vi "S to T - 4Port.vi"(8 "error in (no error)":errorcluster, 11 "S-par Array In":cdb[][](array[numeric])) -> (0 "error out":errorcluster, 3 "T-par Array Out":cdb[][](array[numeric]))   [LabVIEW 2020]
uses:
  <vilib>/Analysis/Matrix/Datatypes/RealMatrix.ctl
  <vilib>/Analysis/baseanly.llb/Complex A x B.vi
  <vilib>/Analysis/Matrix/Numeric/Conversions/Matrix To Array - RM.vi
  <vilib>/Analysis/Matrix/Numeric/Conversions/Array To Matrix - CA2.vi
  <vilib>/Analysis/Matrix/Numeric/Subtract/Subtract - CM,CM.vi
  <vilib>/addons/HF Network Analysis/NI_HFNetworkAnalysis.lvlib
  <vilib>/Analysis/Matrix/NI_Matrix.lvlib
  <vilib>/Analysis/NI_AALBase.lvlib
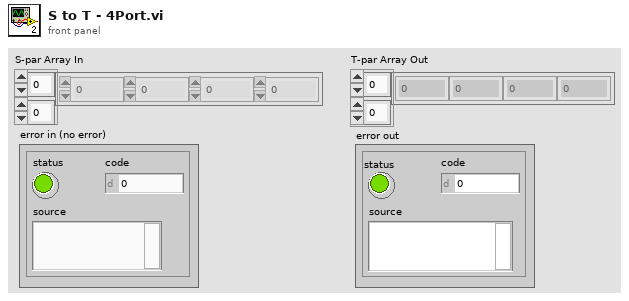
[diagram p1: front panel]
types:
  T1 = typedef "NI_Matrix.lvlib/RealMatrix.ctl" = dbl[][]
  T2 = typedef "NI_Matrix.lvlib/ComplexMatrix.ctl" = cdb[][]
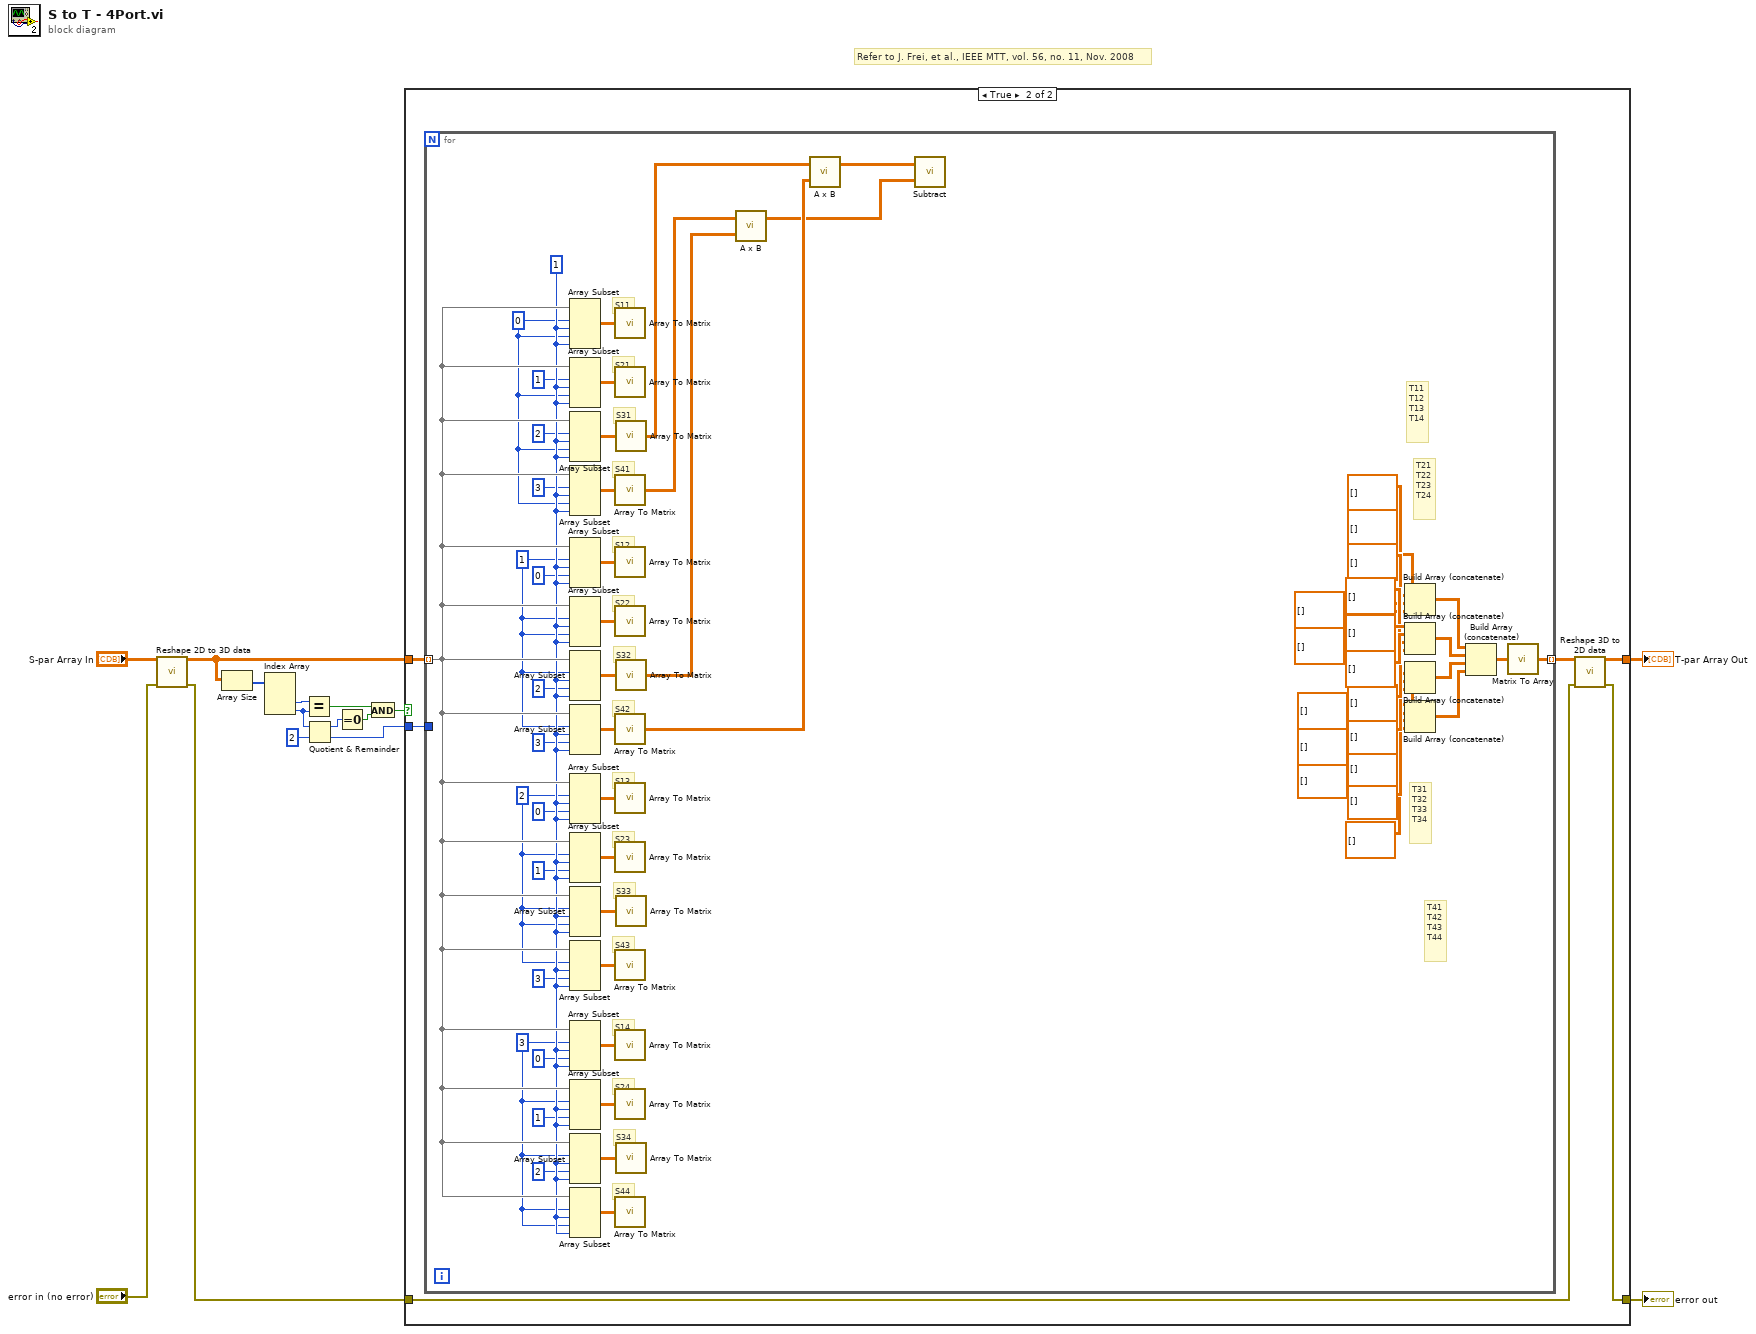
[diagram p0: block diagram]
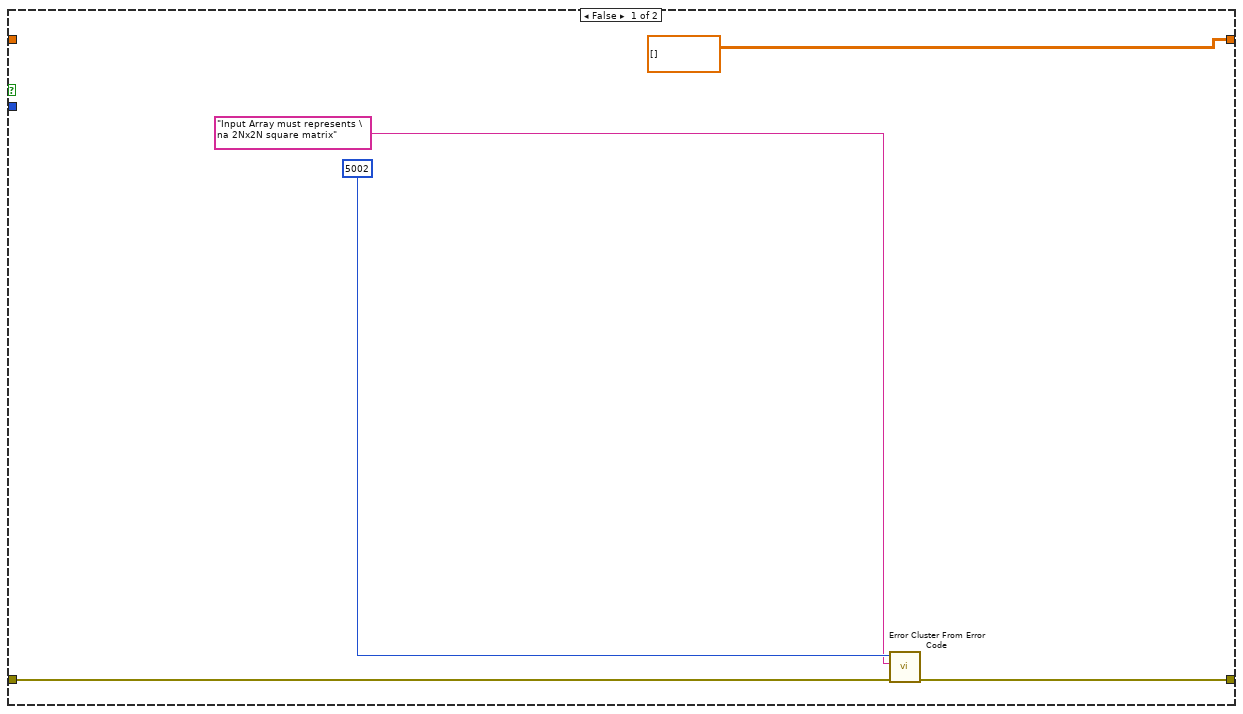
[diagram p2: hidden frame]
diagram:
  # "Refer to J. Frei, et al., IEEE MTT, vol. 56, no. 11, Nov. 2008"
  n1 = call <vilib>:"Reshape 2D to 3D data.vi"("Parameters In (2D)"="S-par Array In", "Error In"="error in (no error)") -> ("Parameters Out (3D)"=w14:cdb[][][], "Error Out"=w5:errorcluster)  [unwired: 12 in]
  n2 = Array Size(array=w14) -> (size(s)=w13:i32[])
  n3 = Index Array(array=w13) -> (element #2=w8:i32, element #3=w12:i32)  [unwired: 3 in, 1 out]
  n4 = Equal?(x=w8, y=w12) -> (x = y?=w10:bool)
  n5 = Quotient & Remainder(x=w12, y=2) -> (x-y*floor(x/y)=w2:i32, floor(x/y)=w1:i32)
  n6 = Equal To 0?(x=w2) -> (x = 0?=w9:bool)
  n7 = And(x=w10, y=w9) -> (x .and. y?=w7:bool)
  n8 = case shown="True" w7 {
    tunnel: w14 -> [_ w26]
    tunnel: w1 -> [_ w25]
    tunnel: [cdb[][] [] ("Parameters Out (2D)") w23] -> w6
    tunnel: w5 -> [w19 w22]
    tunnel: [w18 w21] -> w3
    frame False {
      n9 = call <vilib>:"Error Cluster From Error Code.vi"("error in (no error)"=w19, "error message (\"\")"="Input Array must represents \na 2Nx2N square matrix" ("error message (\"\")"), "error code (0)"=5002) -> ("error out"=w18:errorcluster)  [unwired: 6 in]
    }
    frame True {
      n10 = for {
        tunnel: w26 -> [w68] mode=indexing
        tunnel: w25 -> [_]
        tunnel: [w81] -> w24 mode=indexing
        w60 = 3 ("index")
        w61 = 2 ("index")
        w62 = 1 ("index")
        w66 = 0 ("index")
        w67 = 1 ("length")
        # "T41\nT42\nT43\nT44"
        # "T31\nT32\nT33\nT34"
        # "T21\nT22\nT23\nT24"
        # "T11\nT12\nT13\nT14"
        # "S34"
        # "S44"
        # "S14"
        # "S24"
        # "S33"
        # "S43"
        # "S13"
        # "S23"
        # "S31"
        # "S41"
        # "S11"
        # "S21"
        # "S32"
        # "S42"
        # "S12"
        # "S22"
        n11 = Array Subset(array=w68, index (row)=w66, length (row)=w67, index (col)=w66, length (col)=w67) -> (w78:cdb[][])
        n12 = Array Subset(array=w68, index (row)=1 ("index"), length (row)=w67, index (col)=w66, length (col)=w67) -> (w77:cdb[][])
        n13 = Array Subset(array=w68, index (row)=2 ("index"), length (row)=w67, index (col)=w66, length (col)=w67) -> (w80:cdb[][])
        n14 = Array Subset(array=w68, index (row)=3 ("index"), length (row)=w67, index (col)=w66, length (col)=w67) -> (w79:cdb[][])
        n15 = Array Subset(array=w68, index (row)=w62, length (row)=w67, index (col)=0 ("index"), length (col)=w67) -> (w87:cdb[][])
        n16 = Array Subset(array=w68, index (row)=w62, length (row)=w67, index (col)=w62, length (col)=w67) -> (w88:cdb[][])
        n17 = Array Subset(array=w68, index (row)=w62, length (row)=w67, index (col)=2 ("index"), length (col)=w67) -> (w85:cdb[][])
        n18 = Array Subset(array=w68, index (row)=w62, length (row)=w67, index (col)=3 ("index"), length (col)=w67) -> (w86:cdb[][])
        n19 = Array Subset(array=w68, index (row)=w61, length (row)=w67, index (col)=0 ("index"), length (col)=w67) -> (w75:cdb[][])
        n20 = Array Subset(array=w68, index (row)=w61, length (row)=w67, index (col)=1 ("index"), length (col)=w67) -> (w76:cdb[][])
        n21 = Array Subset(array=w68, index (row)=w61, length (row)=w67, index (col)=w61, length (col)=w67) -> (w73:cdb[][])
        n22 = Array Subset(array=w68, index (row)=w61, length (row)=w67, index (col)=3 ("index"), length (col)=w67) -> (w74:cdb[][])
        n23 = Array Subset(array=w68, index (row)=w60, length (row)=w67, index (col)=0 ("index"), length (col)=w67) -> (w70:cdb[][])
        n24 = Array Subset(array=w68, index (row)=w60, length (row)=w67, index (col)=1 ("index"), length (col)=w67) -> (w69:cdb[][])
        n25 = Array Subset(array=w68, index (row)=w60, length (row)=w67, index (col)=2 ("index"), length (col)=w67) -> (w72:cdb[][])
        n26 = Array Subset(array=w68, index (row)=w60, length (row)=w67, index (col)=w60, length (col)=w67) -> (w71:cdb[][])
        n27 = call-poly <vilib>:"Array To Matrix.vi"("Complex 2D Array"=w78) -> ()  [unwired: 1 out]
        n28 = call-poly <vilib>:"Array To Matrix.vi"("Complex 2D Array"=w77) -> ()  [unwired: 1 out]
        n29 = call-poly <vilib>:"Array To Matrix.vi"("Complex 2D Array"=w79) -> ("Complex Matrix"=w46:T2)
        n30 = call-poly <vilib>:"Array To Matrix.vi"("Complex 2D Array"=w87) -> ()  [unwired: 1 out]
        n31 = call-poly <vilib>:"Array To Matrix.vi"("Complex 2D Array"=w88) -> ()  [unwired: 1 out]
        n32 = call-poly <vilib>:"Array To Matrix.vi"("Complex 2D Array"=w86) -> ("Complex Matrix"=w47:T2)
        n33 = call-poly <vilib>:"Array To Matrix.vi"("Complex 2D Array"=w75) -> ()  [unwired: 1 out]
        n34 = call-poly <vilib>:"Array To Matrix.vi"("Complex 2D Array"=w76) -> ()  [unwired: 1 out]
        n35 = call-poly <vilib>:"Array To Matrix.vi"("Complex 2D Array"=w74) -> ()  [unwired: 1 out]
        n36 = call-poly <vilib>:"Array To Matrix.vi"("Complex 2D Array"=w70) -> ()  [unwired: 1 out]
        n37 = call-poly <vilib>:"Array To Matrix.vi"("Complex 2D Array"=w69) -> ()  [unwired: 1 out]
        n38 = call-poly <vilib>:"Array To Matrix.vi"("Complex 2D Array"=w71) -> ()  [unwired: 1 out]
        n39 = call-poly <vilib>:"Array To Matrix.vi"("Complex 2D Array"=w80) -> ("Complex Matrix"=w48:T2)
        n40 = call-poly <vilib>:"Array To Matrix.vi"("Complex 2D Array"=w85) -> ("Complex Matrix"=w45:T2)
        n41 = call-poly <vilib>:"Array To Matrix.vi"("Complex 2D Array"=w73) -> ()  [unwired: 1 out]
        n42 = call-poly <vilib>:"Array To Matrix.vi"("Complex 2D Array"=w72) -> ()  [unwired: 1 out]
        n43 = call-poly <vilib>:"A x B.vi"("B"=w45, "A"=w46) -> ("A x B"=w43:T2)  [unwired: 1 out]
        n44 = call-poly <vilib>:"A x B.vi"("B"=w47, "A"=w48) -> ("A x B"=w44:T2)  [unwired: 1 out]
        n45 = call-poly <vilib>:"Subtract.vi"("Complex Matrix B"=w43, "Complex Matrix A"=w44) -> ()  [unwired: 1 out]
        n46 = Build Array (concatenate)(T1 [] ("array"), T1 [] ("array"), T1 [] ("array"), T1 [] ("array")) -> (w49:T1)
        n47 = Build Array (concatenate)(T1 [] ("array"), T1 [] ("array"), T1 [] ("array"), T1 [] ("array")) -> (w84:T1)
        n48 = Build Array (concatenate)(T1 [] ("array"), T1 [] ("array"), T1 [] ("array"), T1 [] ("array")) -> (w83:T1)
        n49 = Build Array (concatenate)(T1 [] ("array"), T1 [] ("array"), T1 [] ("array"), T1 [] ("array")) -> (w50:T1)
        n50 = Build Array (concatenate)(w49, w84, w83, w50) -> (w82:T1)
        n51 = call-poly <vilib>:"Matrix To Array.vi"("Real Matrix"=w82) -> ("Real 2D Array"=w81:dbl[][])
      }
      n52 = call <vilib>:"Reshape 3D to 2D data.vi"("Parameters In (3D)"=w24, "Error In"=w22) -> ("Parameters Out (2D)"=w23:cdb[][], "Error Out"=w21:errorcluster)  [unwired: 12 in]
    }
  }
  "T-par Array Out" <- w6
  "error out" <- w3
